vi "On Load.vi"(8 "error in":errorcluster, 11 "Device Item Ref in":T1 format="%.0x") -> (0 "error out":errorcluster, 3 "Device Item Ref out":T1 format="%.0x")   [LabVIEW 2014, in "Scriptable Model Interface System Explorer.lvlib"]
uses:
  Scriptable Model Interface System Explorer.lvlib
  Shared/model inputs.ctl
  Shared/Scriptable Model Interface Shared.lvlib
  Shared/model outputs.ctl
  Shared/model parameters.ctl
  <vilib>/NI Veristand/Custom Device API/Custom Device API.lvlib
  <vilib>/NI Veristand/Custom Device Tools/Custom Device Utility Library/Custom Device Utility Library.lvlib
  <vilib>/NI Veristand/Custom Device API/Custom Device Channel Type.ctl
  Shared/Constants.vi
  <vilib>/NI Veristand/Custom Device API/Set Item Property (String).vi
  <vilib>/NI Veristand/Custom Device API/Get Item Property (String).vi
  <vilib>/NI Veristand/Custom Device API/Custom Device Item Ref.ctl
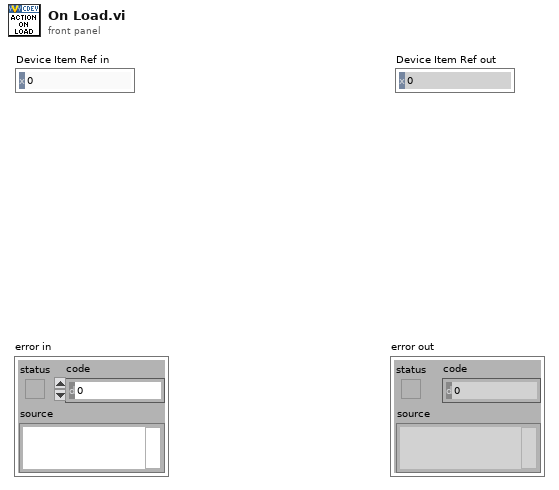
[diagram p1: front panel]
types:
  T1 = typedef "Custom Device API.lvlib/Custom Device Item Ref.ctl" = u64
  T2 = typedef "Custom Device API.lvlib/Custom Device Channel Type.ctl" = enum16{"Input", "Output"}
  T3 = typedef "Scriptable Model Interface Shared.lvlib/model outputs.ctl" = cluster{"o":dbl}
  T4 = typedef "Scriptable Model Interface Shared.lvlib/model inputs.ctl" = cluster{"i":dbl}
  T5 = typedef "Custom Device API.lvlib/Custom Device Channel.ctl" = cluster{"Type":T2, "Units":string, "Default Value":dbl, "Faultable":bool, "Scalable":bool}
  T6 = cluster{"Channel Ref out":T1, "Channel Name":string}
  T7 = typedef "Scriptable Model Interface Shared.lvlib/model parameters.ctl" = cluster{"p":dbl}
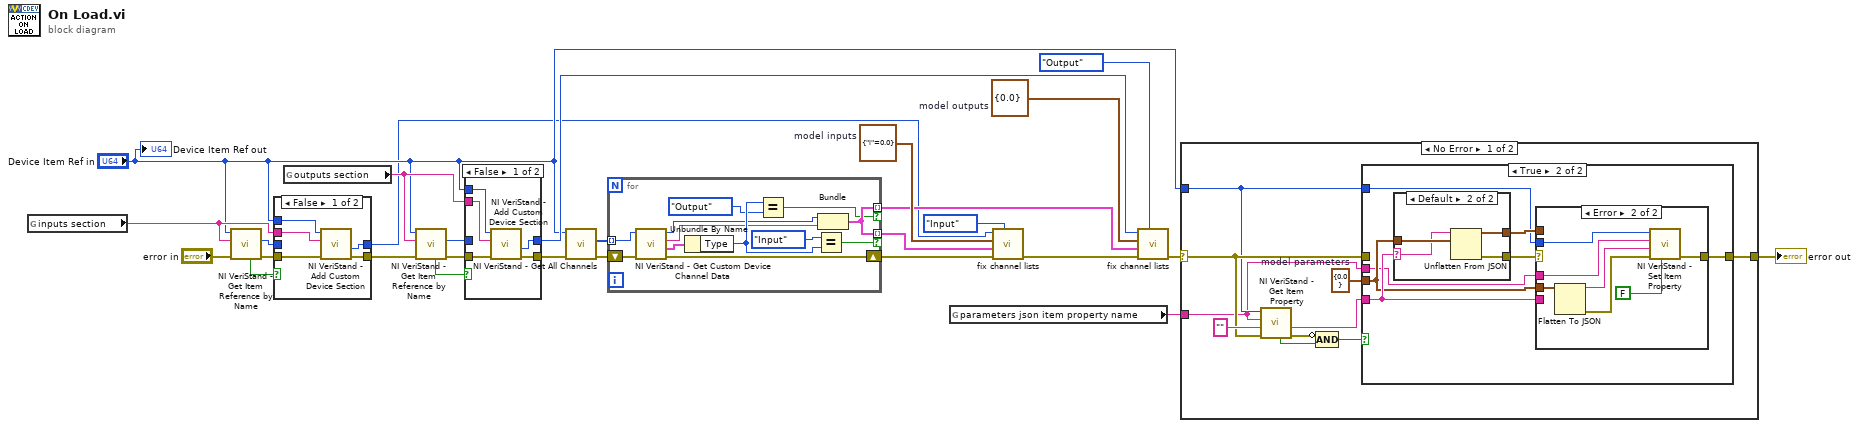
[diagram p0: block diagram]
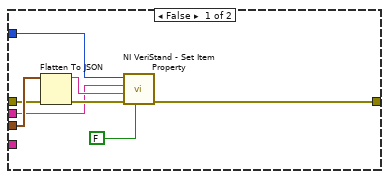
[diagram p4: hidden frame]
diagram:
  w21 = T3 {"o"=0.0}  # model outputs
  w23 = T4 {"i"=0.0}  # model inputs
  n1 = global read "Constants.vi" "inputs section"() -> (w7:string)
  n2 = call <vilib>:"NI VeriStand - Get Item Reference by Name.vi"("error in (no error)"="error in", "Item Name"=w7, "Parent Ref in"="Device Item Ref in") -> ("error out"=w6:errorcluster, "Item Ref"=w3:T1, "Found"=w5:bool)  [unwired: 5 in, 1 out]
  n3 = case shown="False" w5 {
    tunnel: w6 -> [w32 w34]
    tunnel: [w31 w34] -> w4
    tunnel: w7 -> [w30 _]
    tunnel: "Device Item Ref in" -> [w29 _]
    tunnel: [w28 w33] -> w1
    tunnel: w3 -> [_ w33]
    frame False {
      n4 = call <vilib>:"NI VeriStand - Add Custom Device Section.vi"("error in (no error)"=w32, "Section Name"=w30, "Parent Ref in"=w29) -> ("error out"=w31:errorcluster, "Section Ptr"=w28:T1)  [unwired: 5 in, 2 out]
    }
    frame True {
    }
  }
  n5 = global read "Constants.vi" "outputs section"() -> (w10:string)
  n6 = call <vilib>:"NI VeriStand - Get Item Reference by Name.vi"("error in (no error)"=w4, "Item Name"=w10, "Parent Ref in"="Device Item Ref in") -> ("error out"=w12:errorcluster, "Item Ref"=w8:T1, "Found"=w13:bool)  [unwired: 5 in, 1 out]
  n7 = case shown="False" w13 {
    tunnel: w12 -> [w39 w41]
    tunnel: [w38 w41] -> w11
    tunnel: w10 -> [w37 _]
    tunnel: "Device Item Ref in" -> [w36 _]
    tunnel: [w35 w40] -> w9
    tunnel: w8 -> [_ w40]
    frame False {
      n8 = call <vilib>:"NI VeriStand - Add Custom Device Section.vi"("error in (no error)"=w39, "Section Name"=w37, "Parent Ref in"=w36) -> ("error out"=w38:errorcluster, "Section Ptr"=w35:T1)  [unwired: 5 in, 2 out]
    }
    frame True {
    }
  }
  n9 = call <vilib>:"NI VeriStand - Get All Channels.vi"("error in"=w11, "Section Ref in"="Device Item Ref in") -> ("error out"=w27:errorcluster, "Channel Refs"=w26:T1[])  [unwired: 6 in, 2 out]
  n10 = for {
    shift-right: [w52] -> w25
    shift-left: w27 -> [w53]
    tunnel: w26 -> [w51] mode=indexing
    tunnel: [w44] -> w19 mode=indexing if=w43
    tunnel: [w44] -> w18 mode=indexing if=w42
    n11 = call <vilib>:"NI VeriStand - Get Custom Device Channel Data.vi"("error in (no error)"=w53, "Channel Ref in"=w51) -> ("error out"=w52:errorcluster, "Channel"=w50:T5, "Channel Name"=w45:string, "Channel Ref out"=w46:T1)  [unwired: 4 in, 2 out]
    n12 = Unbundle By Name(w50) -> ("Type"=w49:T2)
    n13 = Equal?(x=w49, y=Custom_Device_Channel_Type."Output") -> (x = y?=w42:bool)
    n14 = Equal?(x=Custom_Device_Channel_Type."Input", y=w49) -> (x = y?=w43:bool)
    n15 = Bundle("Channel Ref out"=w46, "Channel Name"=w45) -> (w44:T6)  [unwired: 1 in]
  }
  n16 = global read "Constants.vi" "parameters json item property name"() -> (w15:string)
  n17 = call "fix channel lists.vi"("Type"=Custom_Device_Channel_Type."Input", "error in"=w25, "channels in system definition"=w19, "cluster"=w23, "folder"=w1) -> ("error out"=w22:errorcluster)  [unwired: 6 in]
  n18 = call "fix channel lists.vi"("Type"=Custom_Device_Channel_Type."Output", "error in"=w22, "channels in system definition"=w18, "cluster"=w21, "folder"=w9) -> ("error out"=w17:errorcluster)  [unwired: 6 in]
  n19 = case shown="No Error" w17 {
    selector: w17 -> [w59 w92]
    tunnel: "Device Item Ref in" -> [w58 _]
    tunnel: [w61 w92] -> w16
    tunnel: w15 -> [w57 _]
    frame No Error {
      w60 = T7 {"p"=0.0}  # model parameters
      n20 = call-poly <vilib>:"NI VeriStand - Get Item Property.vi"("error in (no error)"=w59, "Default Value"="", "Property Name"=w57, "Item Ref in"=w58) -> ("error out"=w56:errorcluster, "Value"=w62:string, "Found?"=w55:bool)  [unwired: 4 in, 1 out]
      n21 = Compound Arithmetic op=AND(invert w56, w55) -> (w54:bool)
      n22 = case shown="True" w54 {
        tunnel: w62 -> [_ w75]
        tunnel: [w65 w77] -> w61
        tunnel: w60 -> [w71 w74]
        tunnel: w59 -> [w70 _]
        tunnel: w57 -> [w67 w73]
        tunnel: w58 -> [w66 w72]
        frame False {
          n23 = Flatten To JSON(anything=w71, error in (no error)=w70) -> (JSON string=w68:string, 11:w69:errorcluster)  [unwired: 1 in]
          n24 = call-poly <vilib>:"NI VeriStand - Set Item Property.vi"("Binary String (T)"=FALSE, "error in (no error)"=w69, "Value"=w68, "Property Name"=w67, "Item Ref in"=w66) -> ("error out"=w65:errorcluster)  [unwired: 4 in, 2 out]
        }
        frame True {
          n25 = case shown="Default" w75 {
            selector: w75 -> [_ w88]
            tunnel: [_ w91] -> w78
            tunnel: w74 -> [w87 w90]
            tunnel: [w87 w89] -> w76
            frame "" {
            }
            frame Default {
              n26 = Unflatten From JSON(JSON string=w88, type and defaults=w90) -> (value=w89:T7, error out=w91:errorcluster)  [unwired: 5 in]
            }
          }
          n27 = case shown="Error" w78 {
            selector: w78 -> [w79 _]
            tunnel: [w79 w83] -> w77
            tunnel: w76 -> [_ _]
            tunnel: w75 -> [_ _]
            tunnel: w74 -> [_ w84]
            tunnel: w73 -> [_ w82]
            tunnel: w72 -> [_ w81]
            frame No Error {
            }
            frame Error {
              n28 = Flatten To JSON(anything=w84) -> (JSON string=w85:string, 11:w86:errorcluster)  [unwired: 2 in]
              n29 = call-poly <vilib>:"NI VeriStand - Set Item Property.vi"("Binary String (T)"=FALSE, "error in (no error)"=w86, "Value"=w85, "Property Name"=w82, "Item Ref in"=w81) -> ("error out"=w83:errorcluster)  [unwired: 4 in, 2 out]
            }
          }
        }
      }
    }
    frame Error {
    }
  }
  "error out" <- w16
  "Device Item Ref out" <- "Device Item Ref in"
